vi "Subvi detector change.vi"(7 "Input":bool) -> (1 "Output":bool)   [LabVIEW 2017]
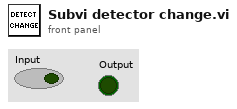
[diagram p1: front panel]
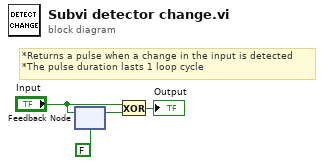
[diagram p0: block diagram]
diagram:
  # "*Returns a pulse when a change in the input is detected\n*The pulse duration lasts 1 loop cycle"
  n1 = feedback-in #1("Input") -> ()
  n2 = feedback #1(FALSE) -> (w4:bool)
  n3 = Exclusive Or(1:w4, 2:"Input") -> (0:→"Output":bool)
